vi "ADC10 LaunchPad.vi"(11 "string":string) -> (2 "ADC10 (Volt)":dbl, 3 "ADCvalue (not convert)":u16)   [LabVIEW 2012]
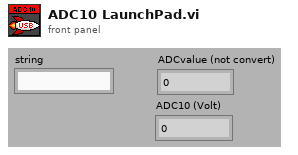
[diagram p1: front panel]
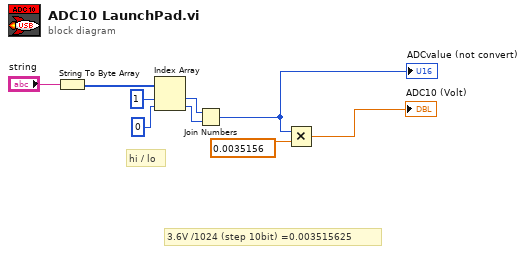
[diagram p0: block diagram]
diagram:
  # "hi / lo"
  # "3.6V /1024 (step 10bit) =0.003515625"
  n1 = String To Byte Array(string="string") -> (unsigned byte array=w1:u8[])
  n2 = Index Array(array=w1, index #1=1 ("index"), index #2=0 ("index")) -> (element #1=w5:u8, element #2=w4:u8)
  n3 = Join Numbers(hi=w5, lo=w4) -> ((hi.lo)=w3:u16)
  "ADCvalue (not convert)" <- w3
  n4 = Multiply(x=w3, y=0.0035156) -> (x*y=→"ADC10 (Volt)":dbl)
